vi "invert_waveform.vi"(9 "invert":bool, 11 "waveform":waveform(dbl)) -> (3 "output waveform":waveform(dbl))   [LabVIEW 2017]
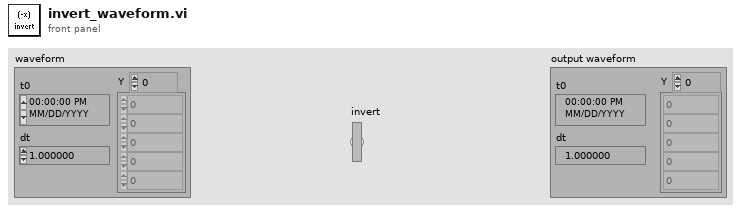
[diagram p1: front panel]
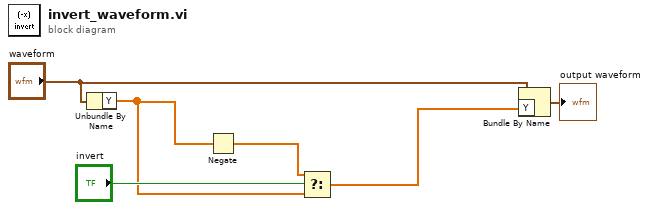
[diagram p0: block diagram]
diagram:
  n1 = Unbundle By Name("waveform") -> ("Y"=w1:dbl[])
  n2 = Negate(x=w1) -> (-x=w2:dbl[])
  n3 = Select(t=w2, s="invert", f=w1) -> (s? t:f=w3:dbl[])
  n4 = Bundle By Name(cluster="waveform", "Y"=w3) -> (→"output waveform":waveform(dbl))
